vi "GPS.vi"(8 "error in (no error)":errorcluster, 10 "reference":refnum<vi>, 11 "VISA Refnum":refnum<visa-resource-name>) -> (0 "error out":errorcluster, 1 "Array":string[](array[string]), 2 "Raw output from GPS":string, 3 "VISA Refnum":refnum<visa-resource-name>, 5 "read buffer":string)   [LabVIEW 2019]
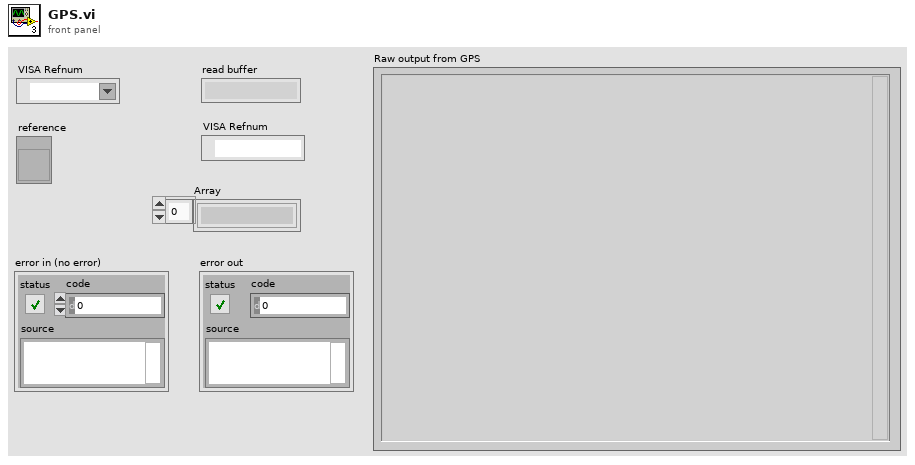
[diagram p1: front panel]
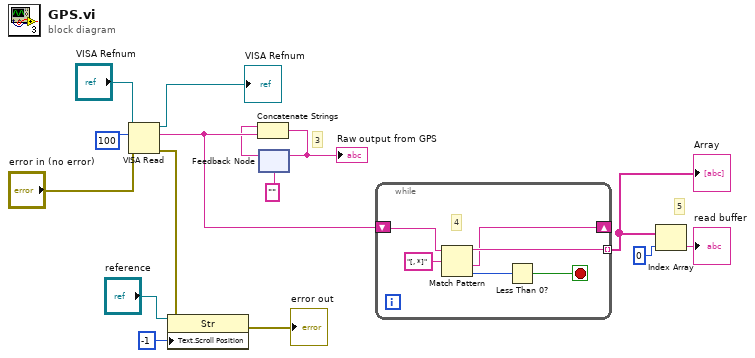
[diagram p0: block diagram]
diagram:
  # "5"
  # "3"
  n1 = VISA Read(VISA resource name="VISA Refnum", byte count=u32 100, error in (no error)="error in (no error)") -> (VISA resource name out=→"VISA Refnum":refnum<visa-resource-name>, read buffer=w6:string, error out=w13:errorcluster)  [unwired: 1 out]
  n2 = property on="Property Node" class="Str"(reference="reference", error in=w13, "Text.Scroll Position"=-1 ("Label.Scroll Position")) -> (error out=→"error out":errorcluster)  [unwired: 1 out]
  n3 = feedback #1("") -> (w4:string)
  n4 = Concatenate Strings(w4, w6) -> (w3:string)
  "Raw output from GPS" <- w3
  n5 = feedback-in #1(w3) -> ()
  n6 = while {
    tunnel: [w19] -> w9 mode=indexing
    shift-right: [w18] -> _
    shift-left: w6 -> [w21]
    stop <- w16 stop-if-true
    # "4"
    n7 = Match Pattern(string=w21, regular expression="[, *]") -> (before substring=w19:string, after substring=w18:string, offset past match=w17:i32)  [unwired: 1 in, 1 out]
    n8 = Less Than 0?(x=w17) -> (x < 0?=w16:bool)
  }
  "Array" <- w9
  n9 = Index Array(array=w9, index=0) -> (element=→"read buffer":string)
